vi "Remove Newest Duplicates.vi"(8 "error in":errorcluster, 11 "XML Document in":refnum<class "XML Document.lvclass">) -> (0 "error out":errorcluster, 3 "XML Document out":refnum<class "XML Document.lvclass">)   [LabVIEW 2014, in "XML Document.lvclass"]
uses:
  XML Document.lvclass
  Node_class/Node.lvclass
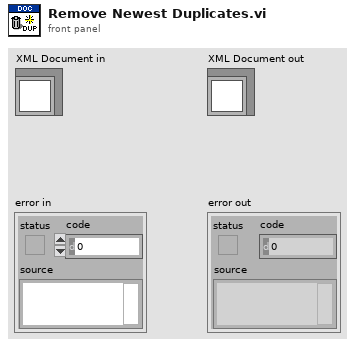
[diagram p1: front panel]
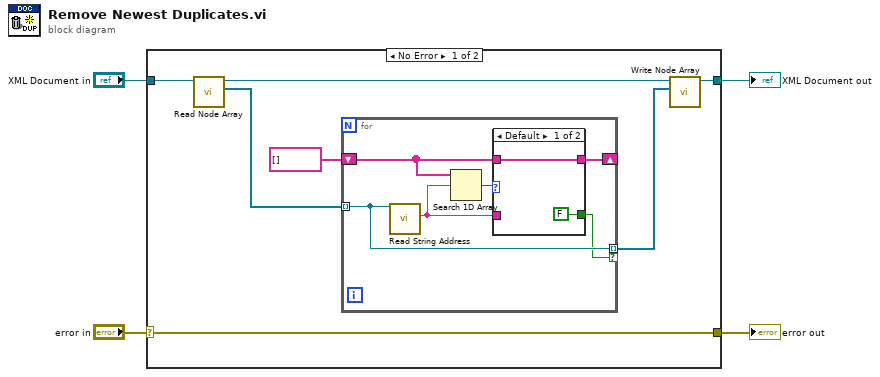
[diagram p0: block diagram]
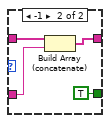
[diagram p2: hidden frame]
diagram:
  n1 = case shown="No Error" "error in" {
    selector: "error in" -> [w10 w25]
    tunnel: [w10 w25] -> w3
    tunnel: [w7 w24] -> w1
    tunnel: "XML Document in" -> [w11 w24]
    frame No Error {
      n2 = call-dynamic "Read Node Array.vi"("XML Document in"=w11) -> ("Node Array"=w6:refnum<class "Node.lvclass">[], "XML Document out"=w8:refnum<class "XML Document.lvclass">)  [unwired: 8 in, 1 out]
      n3 = for {
        tunnel: w6 -> [w13] mode=indexing
        shift-right: [w15] -> _
        shift-left: string[] [] -> [w16]
        tunnel: [w13] -> w5 mode=indexing if=w12
        n4 = call-dynamic "Read String Address.vi"("Node in"=w13) -> ("String Address"=w14:string)  [unwired: 8 in, 2 out]
        n5 = Search 1D Array(1D array=w16, element=w14) -> (index of element=w17:i32)  [unwired: 1 in]
        n6 = case shown="Default" w17 {
          tunnel: w16 -> [w19 w23]
          tunnel: [w19 w21] -> w15
          tunnel: w14 -> [_ w22]
          tunnel: [FALSE TRUE] -> w12
          frame Default {
          }
          frame -1 {
            n7 = Build Array (concatenate)(w23, w22) -> (w21:string[])
          }
        }
      }
      n8 = call-dynamic "Write Node Array.vi"("Node Array"=w5, "XML Document in"=w8) -> ("XML Document out"=w7:refnum<class "XML Document.lvclass">)  [unwired: 8 in, 1 out]
    }
    frame Error {
    }
  }
  "error out" <- w3
  "XML Document out" <- w1
